vi "unused_stackInGrid.vi"(4 "preferredDirection":T2, 5 "alignmentInTheSecondaryDirection":T1, 6 "elementsInPreferredDirection":i32, 7 "useControlBodyOnly":bool, 8 "error in (no error)":errorcluster, 9 "horizontalSpacing":u16, 10 "verticalSpacing":u16, 11 "refs":refnum<vi>[](array[refnum])) -> (0 "error out":errorcluster, 3 "refs(dup)":refnum<vi>[](array[refnum]))   [LabVIEW 2023]
doc: "Stacks the input controls into a structured grid layout.\nArranges the controls using the specified horizontal and vertical spacing. Controls are positioned according to their order in the array.\nThe preferred direction determines whether the grid is filled row-wise (horizontal) or column-wise (vertical).\nThe number of elements in the preferred direction defines the number of columns (if horizontal) or rows (if vertical).\nColumn widths and row heights are determined by the maximum size of the controls within each column or row."
uses:
  direction.ctl
  alignment.ctl
  TLC_Geometry.lvlib
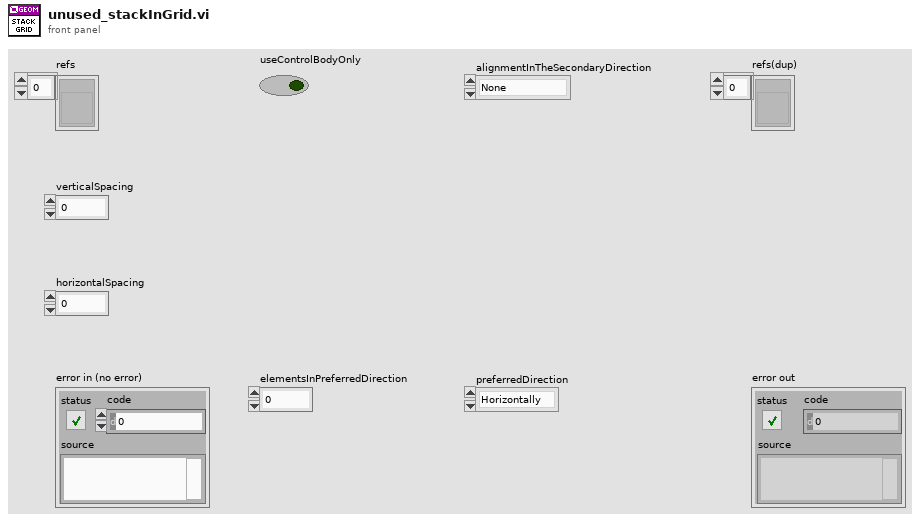
[diagram p1: front panel]
types:
  T1 = typedef "TLC_Geometry.lvlib/alignment.ctl" = enum16{"None", "AlignTop", "AlignBottom", "AlignHorizontalCenters", "AlignLeft", "AlignRight", "AlignVerticalCenters"}
  T2 = typedef "TLC_Geometry.lvlib/direction.ctl" = enum16{"Horizontally", "Vertically"}
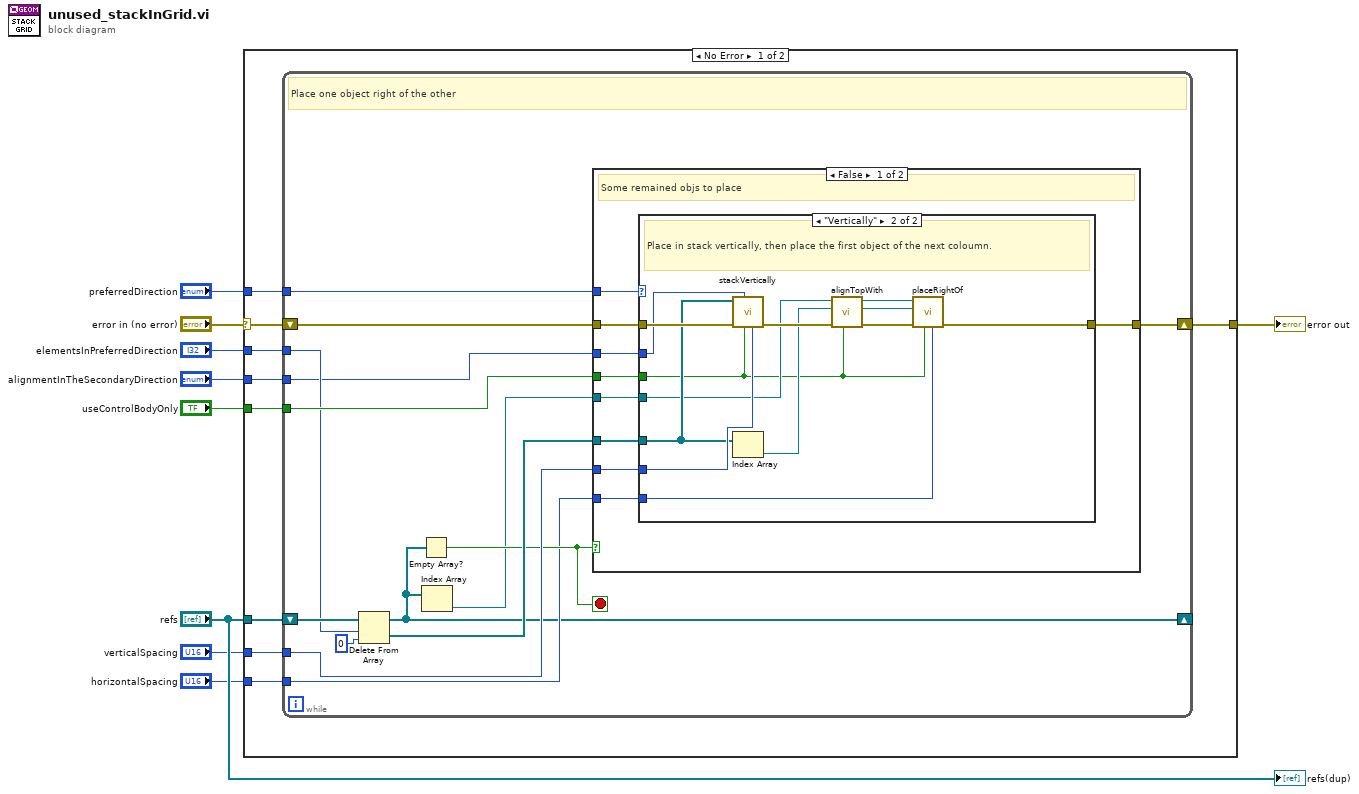
[diagram p0: block diagram]
diagram:
  n1 = case shown="No Error" "error in (no error)" {
    selector: "error in (no error)" -> [w18 w57]
    tunnel: [w17 w57] -> w6
    tunnel: "refs" -> [w13 _]
    tunnel: "useControlBodyOnly" -> [w16 _]
    tunnel: "verticalSpacing" -> [w15 _]
    tunnel: "preferredDirection" -> [w14 _]
    tunnel: "elementsInPreferredDirection" -> [w12 _]
    tunnel: "alignmentInTheSecondaryDirection" -> [w11 _]
    tunnel: "horizontalSpacing" -> [w10 _]
    frame No Error {
      n2 = while {
        shift-right: [w31] -> w17
        shift-left: w18 -> [w32]
        tunnel: w16 -> [w30]
        tunnel: w15 -> [w29]
        tunnel: w14 -> [w28]
        shift-right: [w20] -> _
        shift-left: w13 -> [w27]
        tunnel: w12 -> [w26]
        tunnel: w11 -> [w22]
        tunnel: w10 -> [w21]
        stop <- w23 stop-if-true
        # "Place one object right of the other"
        n3 = Delete From Array(array=w27, length=w26, index=0) -> (deleted portion=w24:refnum<vi>[], array with subset deleted=w20:refnum<vi>[])
        n4 = Empty Array?(array=w20) -> (empty?=w23:bool)
        n5 = Index Array(array=w20) -> (element=w19:refnum<vi>)  [unwired: 1 in]
        n6 = case shown="False" w23 {
          tunnel: w32 -> [w41 w56]
          tunnel: [w40 w56] -> w31
          tunnel: w30 -> [w39 _]
          tunnel: w29 -> [w38 _]
          tunnel: w28 -> [w37 _]
          tunnel: w24 -> [w36 _]
          tunnel: w22 -> [w35 _]
          tunnel: w21 -> [w34 _]
          tunnel: w19 -> [w33 _]
          frame False {
            # "Some remained objs to place"
            n7 = case shown="\"Vertically\"" w37 {
              tunnel: w41 -> [w42 w55]
              tunnel: [w42 w52] -> w40
              tunnel: w39 -> [_ w43]
              tunnel: w38 -> [_ w54]
              tunnel: w36 -> [_ w51]
              tunnel: w35 -> [_ w53]
              tunnel: w34 -> [_ w50]
              tunnel: w33 -> [_ w46]
              frame "Horizontally", Default {
              }
              frame "Vertically" {
                # "Place in stack vertically, then place the first object of the next coloumn."
                n8 = call "stackVertically.vi"("spacing"=w54, "useControlBodyOnly"=w43, "horizontalAlignment"=w53, "error in (no error)"=w55, "refs"=w51) -> ("error out"=w49:errorcluster)  [unwired: 5 in, 1 out]
                n9 = Index Array(array=w51) -> (element=w45:refnum<vi>)  [unwired: 1 in]
                n10 = call "alignTopWith.vi"("useControlBodyOnly"=w43, "error in (no error)"=w49, "anchorObject"=w45, "movingObject"=w46) -> ("error out"=w48:errorcluster, "anchorObject(dup)"=w44:refnum<vi>, "movingObject(dup)"=w47:refnum<vi>)  [unwired: 5 in]
                n11 = call "placeRightOf.vi"("spacing"=w50, "useControlBodyOnly"=w43, "error in (no error)"=w48, "anchorObject"=w44, "movingObject"=w47) -> ("error out"=w52:errorcluster)  [unwired: 4 in, 2 out]
              }
            }
          }
          frame True {
            # "Nothing to do.."
          }
        }
      }
    }
    frame Error {
    }
  }
  "error out" <- w6
  "refs(dup)" <- "refs"
